vi "ElectricalPhase.vi"() -> ()   [LabVIEW 2012]
uses:
  <vilib>/imath/engines/lvmath/Plug In/_Char/NIMS_CH_character datatype.ctl
  <vilib>/Utility/inputDevices.llb/closeKeyboard.vi
  <vilib>/imath/engines/lvmath2/RunTimeEngine/ErrorHandling/NIMS_Finalize Error.vi
  <vilib>/imath/engines/lvmath2/RunTimeEngine/Managers/WorkSpace/UID Generator.vi
  <vilib>/imath/engines/lvmath2/RunTimeEngine/Managers/SymbolTable/Clear UID.vi
  <vilib>/imath/engines/lvmath/Plug In/_Char/NIMS_CH_Character RV to String.vi
  <vilib>/imath/engines/lvmath2/RunTimeEngine/NodeEndStatement/NIMS_NodeEndStatement_Output.vi
  <instcachedir>/0/NIMS_NodeEndStatement_Output_53EC0D466D134D7ABD903AC30B43404B.lvgen/NIMS_NodeEndStatement_Output_53EC0D466D134D7ABD903AC30B43404B_009.vi
  <vilib>/imath/engines/lvmath2/RunTimeEngine/RunTimeType/NIMS_RunTimeType_From StrictType (excl LVString).vi
  <instcachedir>/0/NIMS_RunTimeType_From StrictType (excl LVString)_AC52D965D0864706932D20A05968E122.lvgen/NIMS_RunTimeType_From StrictType (excl LVString)_AC52D965D0864706932D20A05968E122_001.vi
  <vilib>/imath/engines/lvmath2/RunTimeEngine/LocalVariableDefStatement/MC_LocalVariableDefStatement_Display.vi
  <vilib>/Utility/inputDevices.llb/keyboardAcquire.vi
  <vilib>/imath/engines/lvmath2/RunTimeEngine/Managers/SymbolTable/NIMS_WorkSpace.lvlib
panel:
  out "Encoder Value":bool
  out "Bump Sensor":bool
  out "Color Box":u32(colorbox)
  out "Blue":dbl(knob) scale=0.0..100.0
  out "Green":dbl(knob) scale=0.0..100.0
  out "Red":dbl(knob) scale=0.0..100.0
  out "Sonar Volts":dbl
  out "Speed Balance":i32(knob) scale=-600.0..600.0
  out "IR Volts":dbl
  in  "ESTOP":bool
  in  "Step Size":i32=5
  in  "PC Status":i32=1
  in  "Pan Camera":i32(slide)=1500 scale=500.0..2500.0
  out "Starboard Speed":i32(knob) scale=1150.0..1750.0
  out "Port Speed":i32(knob) scale=1150.0..1750.0
  out "Starboard\nMotor":i32
  out "Port\nMotor":i32
  in  "Rudders":i32(slide)=1500 scale=500.0..2500.0
  out "Right Rubber":i32
  out "Left Rudder":i32
  out "String Received":string
  out "return count":u32
  out "bytes written":u32
  out "Blinky":bool
  in  "String":string="$CS1500P1500R1500L1500P1500H   1\n"
  in  "stop":bool
  in  "VISA resource name":refnum<visa-resource-name>="COM7"
  # "ROBOT CONTROL VI\nElectrical Phase for the Roadkill\n\nVPreston\n3/4/2014"
  # "Raw Data"
  # "Motor Control"
  # "Direction of thrust"
  # "Color Panel - Using the little red one"
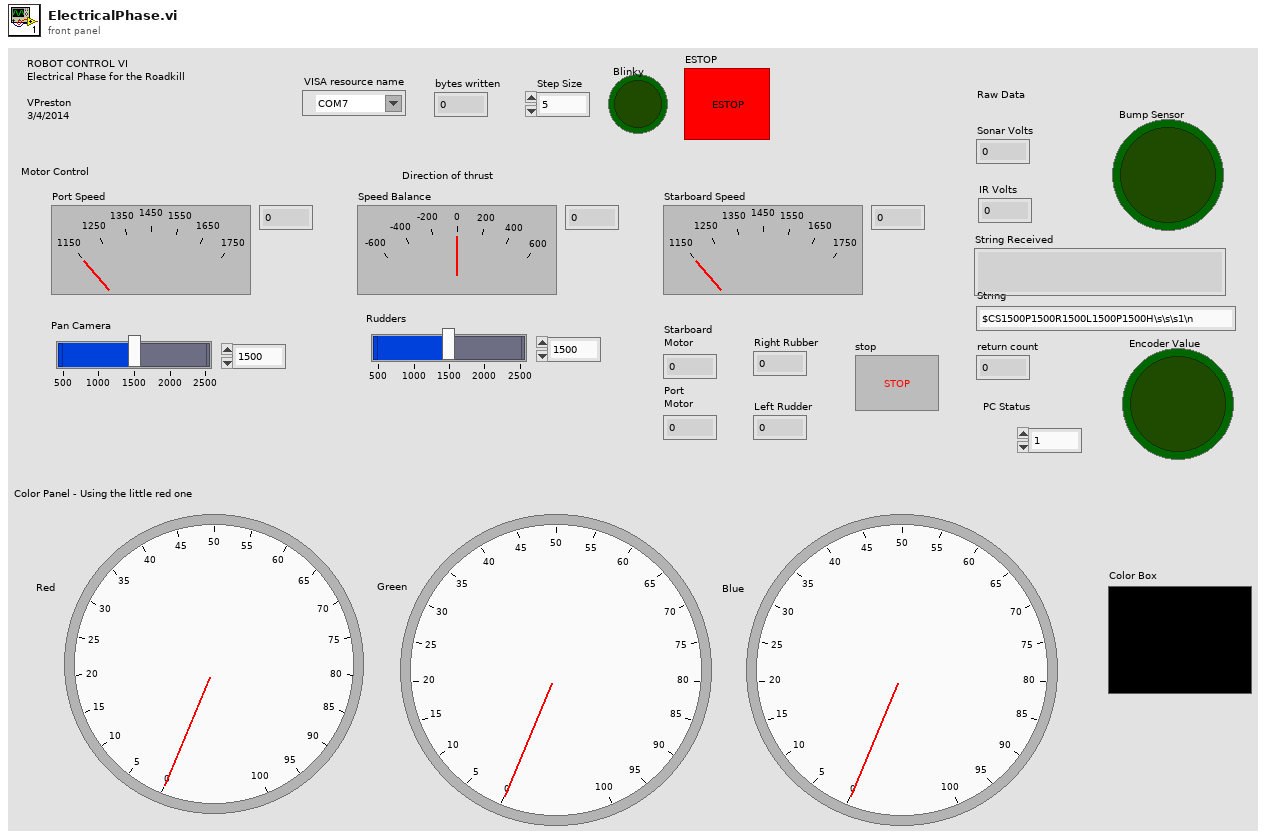
[diagram p1: front panel]
types:
  T1 = enum16{"0", "1", "2", "3", "4", "5", "6", "7", "8", "9", "A", "B", "C", "D", "E", "F", "G", "H", "I", "J", "K", "L", "M", "N", "O", "P", "Q", "R", "S", "T", "U", "V", "W", "X", "Y", "Z", "F1", "F2", "F3", "F4", "F5", "F6", "F7", "F8", "F9", "F10", "F11", "F12", "F13", "F14", "F15", "ADD", "BACK", "BACKSLASH", "CAPITAL", "COMMA", "DECIMAL", "DELETE", "DIVIDE", "DOWN", "END", "EQUALS", "ESCAPE", "GRAVE (`)", "HOME", "INSERT", "LBRACKET", "LCONTROL", "LEFT", "L ALT", "LSHIFT", "LWIN", "MINUS", "MULTIPLY", "NEXT", "NUMLOCK", "NUMPAD_0", "NUMPAD_1", "NUMPAD_2", "NUMPAD_3", "NUMPAD_4", "NUMPAD_5", "NUMPAD_6", "NUMPAD_7", "NUMPAD_8", "NUMPAD_9", "PAUSE", "PERIOD", "PRIOR (PG UP)", "RBRACKET", "RCONTROL", "RETURN", "RIGHT", "R ALT", "RSHIFT", "RWIN", "SCROLL", "SEMICOLON", "SLASH", "SPACE", "SUBTRACT", "TAB", "UP", "ENTER (num pad)", "' (quote)"}[]
  T2 = enum16{"0", "1", "2", "3", "4", "5", "6", "7", "8", "9", "A", "B", "C", "D", "E", "F", "G", "H", "I", "J", "K", "L", "M", "N", "O", "P", "Q", "R", "S", "T", "U", "V", "W", "X", "Y", "Z", "F1", "F2", "F3", "F4", "F5", "F6", "F7", "F8", "F9", "F10", "F11", "F12", "F13", "F14", "F15", "ADD", "BACK", "BACKSLASH", "CAPITAL", "COMMA", "DECIMAL", "DELETE", "DIVIDE", "DOWN", "END", "EQUALS", "ESCAPE", "GRAVE (`)", "HOME", "INSERT", "LBRACKET", "LCONTROL", "LEFT", "L ALT", "LSHIFT", "LWIN", "MINUS", "MULTIPLY", "NEXT", "NUMLOCK", "NUMPAD_0", "NUMPAD_1", "NUMPAD_2", "NUMPAD_3", "NUMPAD_4", "NUMPAD_5", "NUMPAD_6", "NUMPAD_7", "NUMPAD_8", "NUMPAD_9", "PAUSE", "PERIOD", "PRIOR (PG UP)", "RBRACKET", "RCONTROL", "RETURN", "RIGHT", "R ALT", "RSHIFT", "RWIN", "SCROLL", "SEMICOLON", "SLASH", "SPACE", "SUBTRACT", "TAB", "UP", "ENTER (num pad)", "' (quote)"}
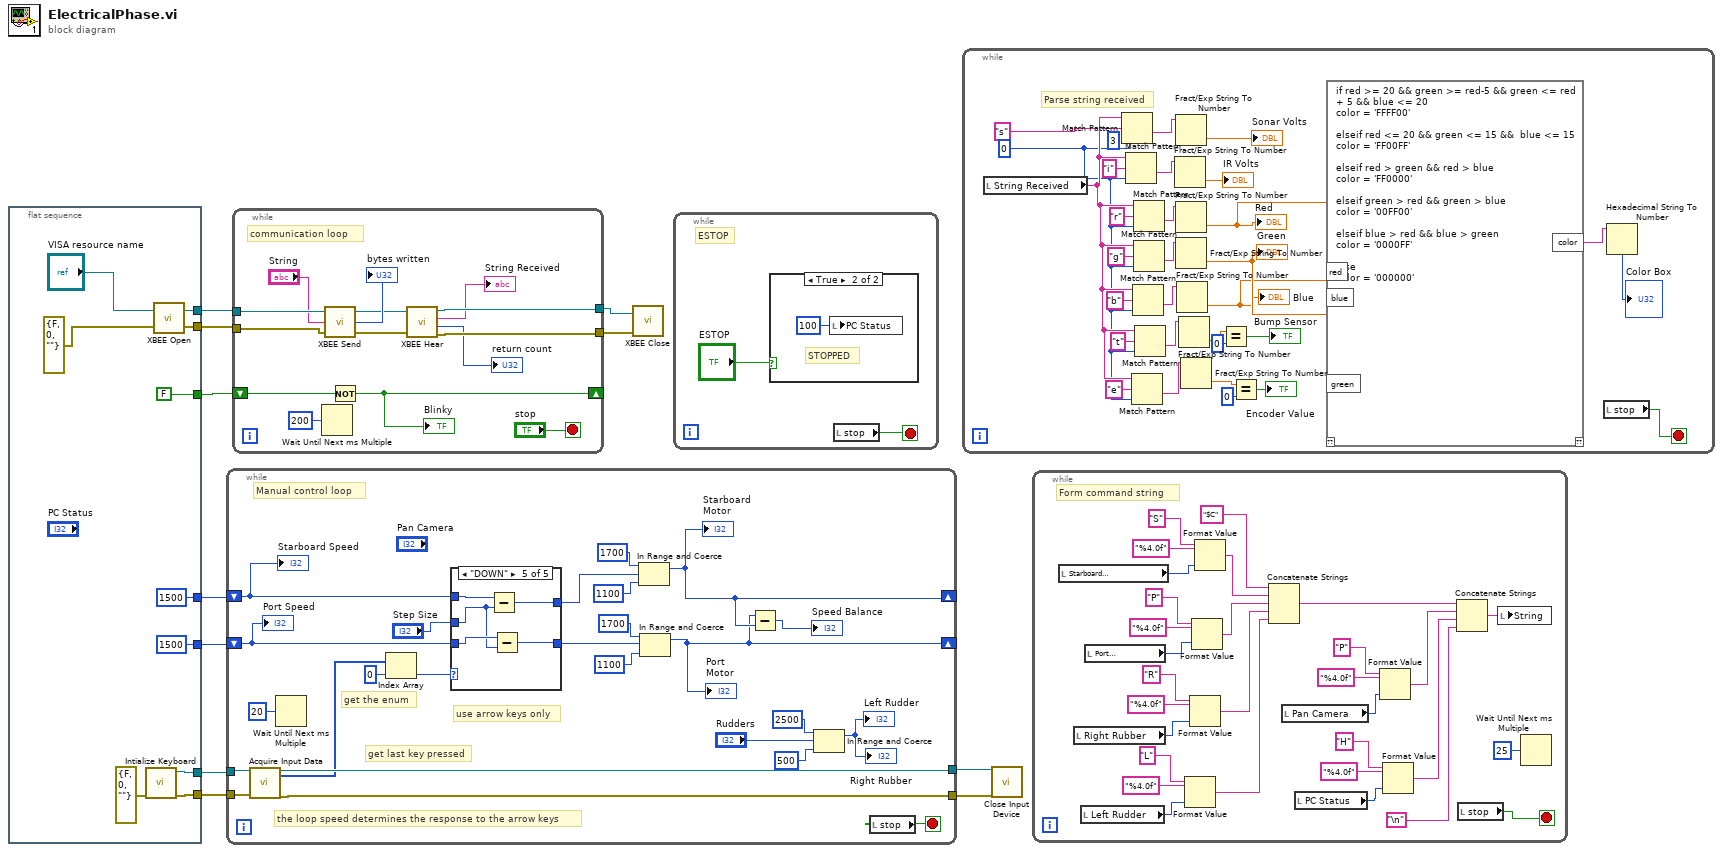
[diagram p0: block diagram]
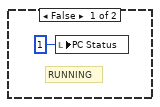
[diagram p2: hidden frame]
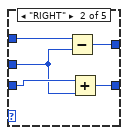
[diagram p4: hidden frame]
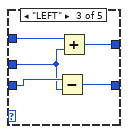
[diagram p5: hidden frame]
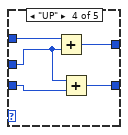
[diagram p6: hidden frame]
diagram:
  n1 = flat-sequence {
    tunnel: [w21] -> w11
    tunnel: [w20] -> w10
    tunnel: [FALSE] -> w7
    tunnel: [w18] -> w6
    tunnel: [w16] -> w5
    tunnel: [1500] -> w2
    tunnel: [1500] -> w1
    frame #0 {
      n2 = call <vilib>:"Intialize Keyboard.vi"("error in (no error)"=errorcluster {"status"=FALSE, "code"=0, "source"=""}) -> ("error out"=w18:errorcluster, "device ID"=w16:refnum<k1>)  [unwired: 9 in]
      n3 = call "XBEE Open.vi"("error in"=errorcluster {"status"=FALSE, "code"=0, "source"=""}, "VISA resource name"="VISA resource name") -> ("error out"=w20:errorcluster, "VISA resource name out"=w21:refnum<visa-resource-name>)
    }
  }
  n4 = while {
    tunnel: w6 -> [w46]
    tunnel: w5 -> [w45]
    tunnel: [w44] -> w4
    tunnel: [w43] -> w3
    shift-right: [w23] -> _
    shift-left: w1 -> [w38]
    shift-right: [w22] -> _
    shift-left: w2 -> [w37]
    stop <- w29 stop-if-true
    # "use arrow keys only"
    # "Manual control loop"
    # "get the enum"
    # "the loop speed determines the response to the arrow keys"
    # "get last key pressed"
    n5 = call-poly <vilib>:"Acquire Input Data.vi"("device ID"=w45, "error in (no error)"=w46) -> ("device ID"=w43:refnum<k1>, "keys pressed"=w42:T1, "error out"=w44:errorcluster)  [unwired: 15 in]
    n6 = Wait Until Next ms Multiple(millisecond multiple=u32 20) -> ()  [unwired: 1 out]
    n7 = Index Array(array=w42, index=0) -> (element=w40:T2)
    n8 = case shown="\"DOWN\"" w40 {
      tunnel: w38 -> [w48 w50 w55 w63 w68]
      tunnel: [w48 w51 w56 w62 w67] -> w36
      tunnel: w37 -> [w47 w53 w57 w60 w66]
      tunnel: [w47 w52 w58 w59 w64] -> w25
      tunnel: "Step Size" -> [_ w49 w54 w61 w65]
      frame "0", Default {
      }
      frame "RIGHT" {
        n9 = Subtract(x=w50, y=w49) -> (x-y=w51:i32)
        n10 = Add(x=w53, y=w49) -> (x+y=w52:i32)
      }
      frame "LEFT" {
        n11 = Subtract(x=w57, y=w54) -> (x-y=w58:i32)
        n12 = Add(x=w55, y=w54) -> (x+y=w56:i32)
      }
      frame "UP" {
        n13 = Add(x=w63, y=w61) -> (x+y=w62:i32)
        n14 = Add(x=w61, y=w60) -> (x+y=w59:i32)
      }
      frame "DOWN" {
        n15 = Subtract(x=w68, y=w65) -> (x-y=w67:i32)
        n16 = Subtract(x=w66, y=w65) -> (x-y=w64:i32)
      }
    }
    n17 = In Range and Coerce(upper limit=1700, x=w36, lower limit=1100) -> (coerced(x)=w23:i32)  [unwired: 1 out]
    "Starboard\nMotor" <- w23
    n18 = In Range and Coerce(upper limit=1700, x=w25, lower limit=1100) -> (coerced(x)=w22:i32)  [unwired: 1 out]
    "Port\nMotor" <- w22
    n19 = Subtract(x=w22, y=w23) -> (x-y=→"Speed Balance":i32)
    n20 = In Range and Coerce(upper limit=2500, x="Rudders", lower limit=500) -> (coerced(x)=→"Right Rubber" →"Left Rudder":i32)  [unwired: 1 out]
    n21 = local read "stop"() -> (w29:bool)
    "Starboard Speed" <- w38
    "Port Speed" <- w37
  }
  n22 = while {
    tunnel: w11 -> [w81]
    tunnel: w10 -> [w80]
    tunnel: [w75] -> w9
    tunnel: [w74] -> w8
    shift-right: [w78] -> _
    shift-left: w7 -> [w79]
    stop <- "stop" stop-if-true
    # "communication loop"
    n23 = Wait Until Next ms Multiple(millisecond multiple=u32 200) -> ()  [unwired: 1 out]
    n24 = call "XBEE Send.vi"("error in (no error)"=w80, "String"="String", "VISA resource name"=w81) -> ("error out"=w71:errorcluster, "return count"=→"bytes written":u32, "VISA resource name out"=w72:refnum<visa-resource-name>)
    n25 = Not(x=w79) -> (.not. x?=w78:bool)
    "Blinky" <- w78
    n26 = call "XBEE Hear.vi"("VISA resource name"=w72, "error in (no error)"=w71) -> ("VISA resource name out"=w75:refnum<visa-resource-name>, "String Received"=→"String Received":string, "return count"=→"return count":u32, "error out"=w74:errorcluster)
  }
  n27 = call "XBEE Close.vi"("error in (no error)"=w8, "VISA resource name"=w9) -> ()
  n28 = while {
    stop <- w84 stop-if-true
    # "ESTOP"
    n29 = case shown="True" "ESTOP" {
      frame False {
        # "RUNNING"
        n30 = local write "PC Status"(1 ("PC Status")) -> ()
      }
      frame True {
        # "STOPPED"
        n31 = local write "PC Status"(100) -> ()
      }
    }
    n32 = local read "stop"() -> (w84:bool)
  }
  n33 = while {
    stop <- w116 stop-if-true
    (unwired) 3 ("offset past match")
    w99 = 0 ("offset (0)")
    # "Parse string received"
    n34 = local read "String Received"() -> (w101:string)
    n35 = Match Pattern(string=w101, regular expression="s", offset (0)=w99) -> (after substring=w102:string)  [unwired: 3 out]
    n36 = Match Pattern(string=w101, regular expression="i", offset (0)=w99) -> (after substring=w92:string)  [unwired: 3 out]
    n37 = Match Pattern(string=w101, regular expression="e", offset (0)=w99) -> (after substring=w87:string)  [unwired: 3 out]
    n38 = Match Pattern(string=w101, regular expression="b", offset (0)=w99) -> (after substring=w89:string)  [unwired: 3 out]
    n39 = Match Pattern(string=w101, regular expression="r", offset (0)=w99) -> (after substring=w91:string)  [unwired: 3 out]
    n40 = Match Pattern(string=w101, regular expression="g", offset (0)=w99) -> (after substring=w90:string)  [unwired: 3 out]
    n41 = Match Pattern(string=w101, regular expression="t", offset (0)=w99) -> (after substring=w88:string)  [unwired: 3 out]
    n42 = Fract/Exp String To Number(string=w92) -> (number=→"IR Volts":dbl)  [unwired: 3 in, 1 out]
    n43 = Fract/Exp String To Number(string=w102) -> (number=→"Sonar Volts":dbl)  [unwired: 3 in, 1 out]
    n44 = Fract/Exp String To Number(string=w91) -> (number=w113:dbl)  [unwired: 3 in, 1 out]
    "Red" <- w113
    n45 = Fract/Exp String To Number(string=w90) -> (number=w112:dbl)  [unwired: 3 in, 1 out]
    "Green" <- w112
    n46 = Fract/Exp String To Number(string=w89) -> (number=w111:dbl)  [unwired: 3 in, 1 out]
    "Blue" <- w111
    n47 = Fract/Exp String To Number(string=w88) -> (number=w108:dbl)  [unwired: 3 in, 1 out]
    n48 = Fract/Exp String To Number(string=w87) -> (number=w104:dbl)  [unwired: 3 in, 1 out]
    n49 = Equal?(x=w108, y=0) -> (x = y?=→"Bump Sensor":bool)
    n50 = Equal?(x=w104, y=0) -> (x = y?=→"Encoder Value":bool)
    n51 = mathscript code="if red >= 20 && green >= red-5 && green <= red + 5 && blue <= 20\ncolor = 'FFFF00'\n\nelseif red <= 20 && green <= 15 &&  blue <= 15\ncolor = 'FF00FF'\n\nelseif red > green && red > blue\ncolor = 'FF0000'\n\nelseif green > red && green > blue\ncolor = '00FF00'\n\nelseif blue > red && blue > green\ncolor = '0000FF' \n\nelse\ncolor = '000000'\n\nend"("red"=w113, "blue"=w111, "green"=w112) -> ("color"=w110:string)  [unwired: 1 in, 1 out]
    n52 = local read "stop"() -> (w116:bool)
    n53 = Hexadecimal String To Number(string=w110) -> (number=→"Color Box":u32)  [unwired: 2 in, 1 out]
  }
  n54 = call-poly <vilib>:"Close Input Device.vi"("error in (no error)"=w4, "device ID"=w3) -> ()  [unwired: 8 in, 1 out]
  n55 = while {
    stop <- w387 stop-if-true
    # "Form command string"
    n56 = local read "Starboard\nMotor"() -> (w384:i32)
    n57 = local read "Right Rubber"() -> (w375:i32)
    n58 = local read "Left Rudder"() -> (w372:i32)
    n59 = local read "Port\nMotor"() -> (w381:i32)
    n60 = Format Value(string ("")="L", format string="%4.0f", value (0)=w372) -> (output string=w370:string)
    n61 = Format Value(string ("")="R", format string="%4.0f", value (0)=w375) -> (output string=w371:string)
    n62 = Format Value(string ("")="P", format string="%4.0f", value (0)=w381) -> (output string=w378:string)
    n63 = Format Value(string ("")="S", format string="%4.0f", value (0)=w384) -> (output string=w379:string)
    n64 = Concatenate Strings("$C", w379, w378, w371, w370) -> (w362:string)
    n65 = local read "Pan Camera"() -> (w366:i32)
    n66 = local read "PC Status"() -> (w363:i32)
    n67 = Format Value(string ("")="P", format string="%4.0f", value (0)=w366) -> (output string=w361:string)
    n68 = Format Value(string ("")="H", format string="%4.0f", value (0)=w363) -> (output string=w360:string)
    n69 = Concatenate Strings(w362, w361, w360, "\n") -> (w367:string)
    n70 = local read "stop"() -> (w387:bool)
    n71 = local write "String"(w367) -> ()
    n72 = Wait Until Next ms Multiple(millisecond multiple=u32 25) -> ()  [unwired: 1 out]
  }
